vi "Clear Logger.vi"(8 "error in (no error)":errorcluster, 11 "Logger Level in":refnum<class "Logger Level.lvclass">) -> (0 "error out":errorcluster, 3 "Logger Level out":refnum<class "Logger Level.lvclass">)   [LabVIEW 2020, in "Logger Level.lvlib" / "Logger Level.lvclass"]
uses:
  Logger Level.lvclass
  Logger Level Messages/Clear Msg/Clear Msg.lvclass
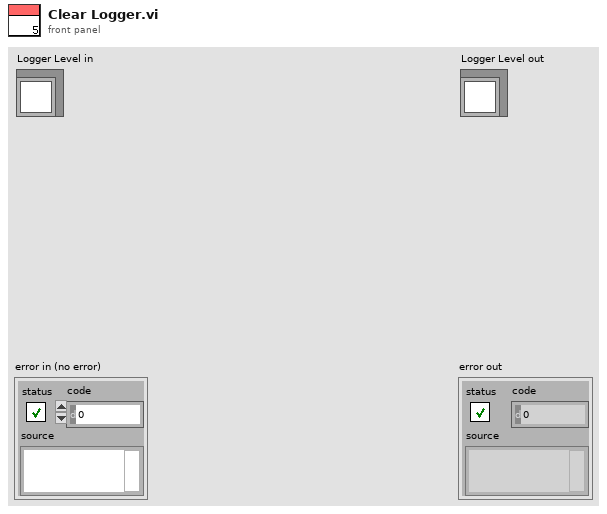
[diagram p1: front panel]
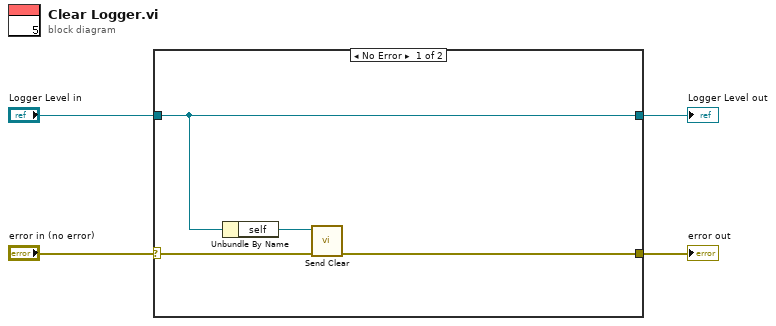
[diagram p0: block diagram]
diagram:
  n1 = case shown="No Error" "error in (no error)" {
    selector: "error in (no error)" -> [w7 w10]
    tunnel: "Logger Level in" -> [w8 w9]
    tunnel: [w5 w10] -> w2
    tunnel: [w8 w9] -> w1
    frame No Error {
      n2 = Unbundle By Name(w8) -> ("self"=w6:refnum<class "Message Enqueuer.lvclass">)
      n3 = call "Send Clear.vi"("error in (no error)"=w7, "Message Enqueuer"=w6) -> ("error out"=w5:errorcluster)  [unwired: 8 in, 1 out]
    }
    frame Error {
    }
  }
  "error out" <- w2
  "Logger Level out" <- w1
